vi "ParseOutputs.vi"(8 "error in (no error)":errorcluster, 9 "Operation Output/Error In":string, 11 "DiscoverTestCases in":refnum<class "DiscoverTestCases.lvclass">) -> (0 "error out":errorcluster, 1 "Operation Output/Error Out":string, 2 "CLI Process Return Code":i32, 3 "DiscoverTestCases out":refnum<class "DiscoverTestCases.lvclass">)   [LabVIEW 2027, in "DiscoverTestCases.lvclass"]
uses:
  DiscoverTestCases.lvclass
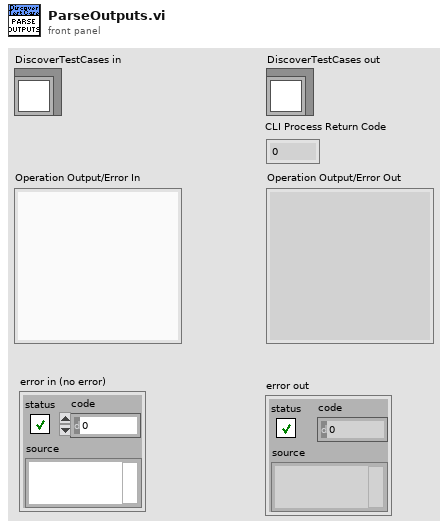
[diagram p1: front panel]
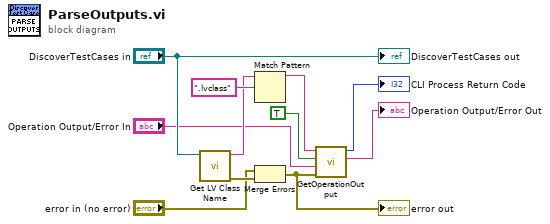
[diagram p0: block diagram]
diagram:
  n1 = call <vilib>:"Get LV Class Name.vi"("object"="DiscoverTestCases in") -> ("error out"=w9:errorcluster, "class name"=w10:string)  [unwired: 9 in]
  n2 = Match Pattern(string=w10, regular expression=".lvclass") -> (before substring=w5:string)  [unwired: 1 in, 3 out]
  n3 = Merge Errors("error in (no error)", w9) -> (w4:errorcluster)
  "error out" <- w4
  n4 = call <nishared>:"GetOperationOutput.vi"("error in (no error)"=w4, "Operation Output/Error In"="Operation Output/Error In", "Operation succeeded?"=TRUE, "Operation Name"=w5) -> ("Operation Output/Error Out"=→"Operation Output/Error Out":string, "CLI Process Return Code"=→"CLI Process Return Code":i32)  [unwired: 6 in]
  "DiscoverTestCases out" <- "DiscoverTestCases in"
